vi "Reserved Names List.vi"() -> (3 "reserved names":string[](array[string])=["MeasurementService Editor", "MeasurementLink Measurement Template", "MeasurementLink Discovery Client", "MeasurementLink Measurement Server", "MeasurementLink Measurement Server Internal", "MeasurementLink Pin Map Client", "MeasurementLink Session Management Client", "grpc-lvsupport-release", "gRPC-servicer-release", "gRPC Template Creation Utility-release", "Client Template", "Service Template"])   [LabVIEW 2021, in "Create Measurement Plug-In Client.lvlib"]
uses:
  Create Measurement Plug-In Client.lvlib
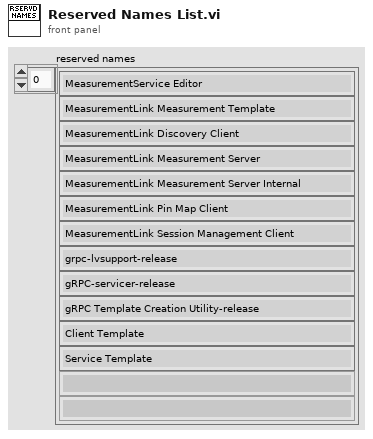
[diagram p1: front panel]
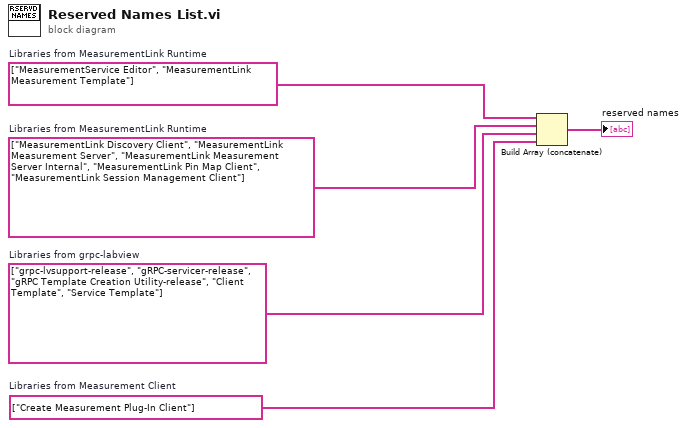
[diagram p0: block diagram]
diagram:
  w1 = string[] ["Create Measurement Plug-In Client"]  # Libraries from Measurement Client
  w3 = string[] ["MeasurementService Editor", "MeasurementLink Measurement Template"]  # Libraries from MeasurementLink Runtime
  w5 = string[] ["grpc-lvsupport-release", "gRPC-servicer-release", "gRPC Template Creation Utility-release", "Client Template", "Service Template"]  # Libraries from grpc-labview
  w4 = string[] ["MeasurementLink Discovery Client", "MeasurementLink Measurement Server", "MeasurementLink Measurement Server Internal", "MeasurementLink Pin Map Client", "MeasurementLink Session Management Client"]  # Libraries from MeasurementLink Runtime
  n1 = Build Array (concatenate)(w3, w4, w5, w1) -> (→"reserved names":string[])
